vi "MGCC_StaEst_funDSE_sub2.vi"(0 "joc_c":dbl[][](array[numeric]), 1 "Ginv":dbl[][](array[numeric]), 2 "joc_d":dbl[][](array[numeric]), 3 "equ_c":dbl[](array[numeric]), 4 "Num":T1, 5 "equ_d":dbl[](array[numeric]), 6 "G2":dbl[](array[numeric])) -> (7 "deltaX":dbl[][](array[numeric]), 8 "tol_temp":dbl[](array[numeric]))   [LabVIEW 2016]
uses:
  <vilib>/imath/engines/lvmath2/RunTimeEngine/RunTimeType/NIMS_RunTimeType_From StrictType (excl LVString).vi
  <instcachedir>/0/NIMS_RunTimeType_From StrictType (excl LVString)_BBF44FB49F834B71AF7A14CCEDF8BECD.lvgen/NIMS_RunTimeType_From StrictType (excl LVString)_BBF44FB49F834B71AF7A14CCEDF8BECD_032.vi
  <instcachedir>/0/NIMS_RunTimeType_From StrictType (excl LVString)_BBF44FB49F834B71AF7A14CCEDF8BECD.lvgen/NIMS_RunTimeType_From StrictType (excl LVString)_BBF44FB49F834B71AF7A14CCEDF8BECD_031.vi
  <vilib>/imath/engines/lvmath2/RunTimeEngine/Struct/NIMS_StructSetField.vi
  <vilib>/imath/engines/lvmath2/RunTimeEngine/Struct/NIMS_StructGetField.vi
  <vilib>/imath/engines/lvmath2/RunTimeEngine/RunTimeType/NIMS_RunTimeType_To Numeric.vi
  <instcachedir>/0/NIMS_RunTimeType_To Numeric_19D51BCABB82435A94073491761E42EE.lvgen/NIMS_RunTimeType_To Numeric_19D51BCABB82435A94073491761E42EE_009.vi
  <instcachedir>/0/NIMS_RunTimeType_To Numeric_19D51BCABB82435A94073491761E42EE.lvgen/NIMS_RunTimeType_To Numeric_19D51BCABB82435A94073491761E42EE_008.vi
  <vilib>/imath/engines/lvmath2/RunTimeEngine/MatrixToken/NIMS_MatrixToken_M_M.vi
  <instcachedir>/0/NIMS_MatrixToken_M_M_DF273B0CC20F424BBF1EDA9F4E71C841.lvgen/NIMS_MatrixToken_M_M_DF273B0CC20F424BBF1EDA9F4E71C841_004.vi
  <vilib>/imathl/engines/lvmath/Functions/Error Handling/Create Error.vi
  <vilib>/imath/engines/lvmath2/RunTimeEngine/RangeToken/NIMS_Range.vi
  <instcachedir>/0/NIMS_Range_A7C094595B484CA7AF10685B02D808ED.lvgen/NIMS_Range_A7C094595B484CA7AF10685B02D808ED_000.vi
  <vilib>/imath/engines/lvmath2/RunTimeEngine/IndexReplace/NIMS M($,V)=S.vi
  <instcachedir>/0/NIMS M($,V)=S_8FF4B0FF94A24B3598424F2A899DBD06.lvgen/NIMS M($,V)=S_8FF4B0FF94A24B3598424F2A899DBD06_000.vi
  <vilib>/imath/engines/lvmath2/RunTimeSupport/NIMS_Error if Not Equal.vi
  <instcachedir>/0/NIMS_Error if Not Equal_43252A79AD05436189442EC0C5E5AB8A.lvgen/NIMS_Error if Not Equal_43252A79AD05436189442EC0C5E5AB8A_001.vi
  <vilib>/imath/engines/lvmath2/RunTimeEngine/ErrorHandling/NIMS_Create Error From Enums.vi
  <vilib>/imath/engines/lvmath2/RunTimeEngine/ArithmeticOperatorToken/NIMS_ArithmeticOperator_multmx.vi
  <instcachedir>/0/NIMS_ArithmeticOperator_multmx_4A56FE5C615140CE835D4DB5891BF065.lvgen/NIMS_ArithmeticOperator_multmx_4A56FE5C615140CE835D4DB5891BF065_004.vi
  <vilib>/imath/engines/lvmath2/RunTimeEngine/BuiltInFunctions/pinv/NIMS_pinv.vi
  <instcachedir>/0/NIMS_pinv_206F0700CF75499C820074BA4F1FFC36.lvgen/NIMS_pinv_206F0700CF75499C820074BA4F1FFC36_000.vi
  <vilib>/imath/engines/lvmath2/RunTimeEngine/ErrorHandling/NIMS_Error From Error Code.vi
  <vilib>/imath/engines/lvmath2/RunTimeEngine/ArithmeticOperatorToken/NIMS_ArithmeticOperator_minus.vi
  <instcachedir>/0/NIMS_ArithmeticOperator_minus_E3B65B1D26A44BB184AFDC5B3F458E3D.lvgen/NIMS_ArithmeticOperator_minus_E3B65B1D26A44BB184AFDC5B3F458E3D_002.vi
  <vilib>/imath/engines/lvmath2/RunTimeEngine/BuiltInFunctions/abs/NIMS_abs(signed).vi
  <instcachedir>/0/NIMS_abs(signed)_C4FCB8E6058B49B797C7C8D53CA5F6EC.lvgen/NIMS_abs(signed)_C4FCB8E6058B49B797C7C8D53CA5F6EC_005.vi
  <vilib>/imath/engines/lvmath2/RunTimeEngine/VariableToken/Support/NIMS_Matrix Boolean Index to I32 Index.vi
  <vilib>/imath/engines/lvmath2/RunTimeEngine/IndexReplace/NIMS M(V)=S.vi
  <instcachedir>/0/NIMS M(V)=S_F2304187E1344F60ABCBE5C5CC0920F9.lvgen/NIMS M(V)=S_F2304187E1344F60ABCBE5C5CC0920F9_000.vi
  <vilib>/imath/engines/lvmath2/RunTimeEngine/BuiltInFunctions/max/1 input/NIMS_max(RM).vi
  <instcachedir>/0/NIMS_max(RM)_358AE92FF7FA4D91BF0D9DEC69043403.lvgen/NIMS_max(RM)_358AE92FF7FA4D91BF0D9DEC69043403_000.vi
  <vilib>/imath/engines/lvmath2/RunTimeEngine/NodeEndStatement/NIMS_NodeEndStatement_Output.vi
  <instcachedir>/0/NIMS_NodeEndStatement_Output_53EC0D466D134D7ABD903AC30B43404B.lvgen/NIMS_NodeEndStatement_Output_53EC0D466D134D7ABD903AC30B43404B_005.vi
  <instcachedir>/0/NIMS_NodeEndStatement_Output_53EC0D466D134D7ABD903AC30B43404B.lvgen/NIMS_NodeEndStatement_Output_53EC0D466D134D7ABD903AC30B43404B_011.vi
  <instcachedir>/0/NIMS_NodeEndStatement_Output_53EC0D466D134D7ABD903AC30B43404B.lvgen/NIMS_NodeEndStatement_Output_53EC0D466D134D7ABD903AC30B43404B_018.vi
  <instcachedir>/0/NIMS_NodeEndStatement_Output_53EC0D466D134D7ABD903AC30B43404B.lvgen/NIMS_NodeEndStatement_Output_53EC0D466D134D7ABD903AC30B43404B_002.vi
  <vilib>/imath/engines/lvmath2/RunTimeEngine/ErrorHandling/NIMS_Finalize Error.vi
panel:
  out "error out":errorcluster
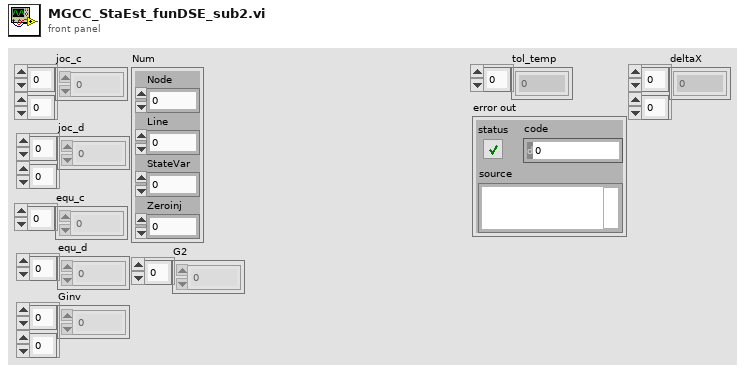
[diagram p1: front panel]
types:
  T1 = cluster{"Node":dbl, "Line":dbl, "StateVar":i32, "Zeroinj":i32}
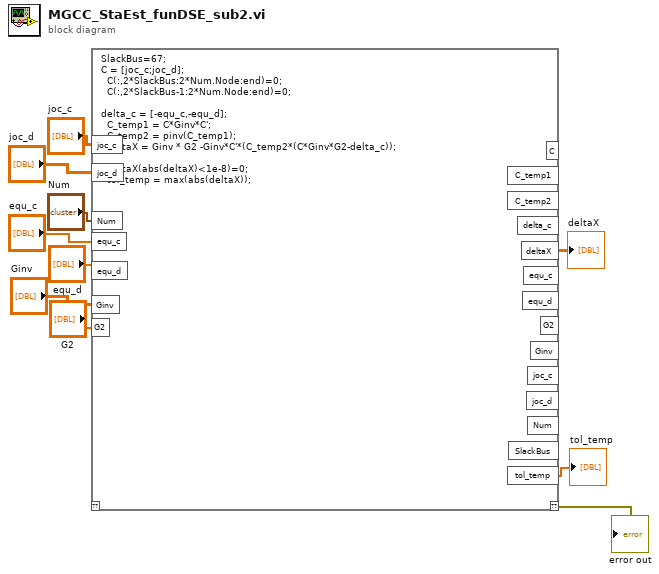
[diagram p0: block diagram]
diagram:
  n1 = mathscript code="SlackBus=67;   \nC = [joc_c;joc_d];\n  C(:,2*SlackBus:2*Num.Node:end)=0;\n  C(:,2*SlackBus-1:2*Num.Node:end)=0;\n\ndelta_c = [-equ_c,-equ_d];  \n  C_temp1 = C*Ginv*C';\n  C_temp2 = pinv(C_temp1);\n  deltaX = Ginv * G2 -Ginv*C'*(C_temp2*(C*Ginv*G2-delta_c)); \n\n  deltaX(abs(deltaX)<1e-8)=0;\n  tol_temp = max(abs(deltaX));"("joc_c"="joc_c", "joc_d"="joc_d", "Num"="Num", "equ_c"="equ_c", "equ_d"="equ_d", "Ginv"="Ginv", "G2"="G2") -> ("??"=→"error out":errorcluster, "deltaX"=→"deltaX":dbl[][], "tol_temp"=→"tol_temp":dbl[])  [unwired: 1 in, 12 out]
